vi "Configure Accelerometer.vi"(7 "Initialize":bool, 10 "data":dbl[](array[numeric]) format="%0.2f", 11 "Sensitivity (mV/g)":dbl=0.3) -> (3 "Angle from horizontal (°)":dbl)   [LabVIEW 2014]
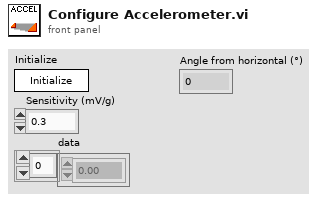
[diagram p1: front panel]
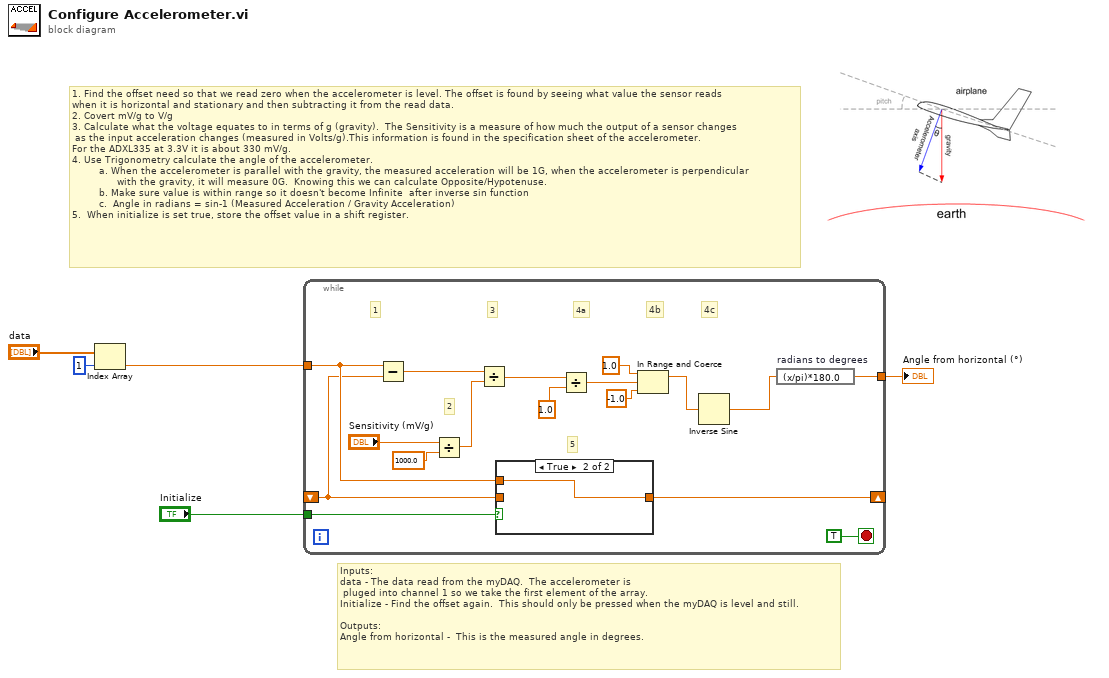
[diagram p0: block diagram]
diagram:
  # "1.\tFind the offset need so that we read zero when the accelerometer is level. The offset is found by seeing what value the sensor reads \nwhen it is horizontal and stationary and then subtracting it from the read data.\n2.\tCovert mV/g to V/g\n3.\tCalculate what the voltage equates to in terms of g (gravity).  The Sensitivity is a measure of how much the output of a sensor changes\n as the input acceleration changes (measured in Volts/g).This information is found in the specification sheet of the accelerometer.  \nFor the ADXL335 at 3.3V it is about 330 mV/g.\n4.\tUse Trigonometry calculate the angle of the accelerometer.\n         a.\tWhen the accelerometer is parallel with the gravity, the measured acceleration will be 1G, when the accelerometer is perpendicular \n               with the gravity, it will measure 0G.  Knowing this we can calculate Opposite/Hypotenuse.\n         b.\tMake sure value is within range so it doesn't become Infinite  after inverse sin function\n         c.\t Angle in radians = sin-1 (Measured Acceleration / Gravity Acceleration)\n5.  When initialize is set true, store the offset value in a shift register."
  # "Inputs:\ndata - The data read from the myDAQ.  The accelerometer is\n pluged into channel 1 so we take the first element of the array.\nInitialize - Find the offset again.  This should only be pressed when the myDAQ is level and still.\n\nOutputs:\nAngle from horizontal -  This is the measured angle in degrees."
  n1 = Index Array(array="data", index=1) -> (element=w1:dbl)
  n2 = while {
    tunnel: w1 -> [w8]
    tunnel: [w13] -> w5
    tunnel: "Initialize" -> [w9]
    shift-right: [w7] -> _
    shift-left: _ -> [w6]
    stop <- TRUE stop-if-true
    # "5"
    # "4c"
    # "4b"
    # "4a"
    # "3"
    # "2"
    # "1"
    n3 = Subtract(x=w8, y=w6) -> (x-y=w22:dbl)
    n4 = Divide(x="Sensitivity (mV/g)", y=1000.0) -> (x/y=w12:dbl)
    n5 = Divide(x=w22, y=w12) -> (x/y=w14:dbl)
    n6 = case shown="True" w9 {
      tunnel: w8 -> [_ w24]
      tunnel: [w23 w24] -> w7
      tunnel: w6 -> [w23 _]
      frame False {
      }
      frame True {
      }
    }
    n7 = Divide(x=w14, y=1.0) -> (x/y=w17:dbl)
    n8 = In Range and Coerce(upper limit=1.0, x=w17, lower limit=-1.0) -> (coerced(x)=w20:dbl)  [unwired: 1 out]
    n9 = Inverse Sine(1:w20) -> (0:w16:dbl)
    n10 = expression code="(x/pi)*180.0" "radians to degrees"(w16) -> (w13:dbl)
  }
  "Angle from horizontal (°)" <- w5
